vi "initialise.vi"(8 "error in (no error)":errorcluster, 10 "main_app_instance":bool, 11 "Pixelfly in":refnum<class "PixelflySA.lvclass">) -> (0 "error out":errorcluster, 3 "Pixelfly out":refnum<class "PixelflySA.lvclass">)   [LabVIEW 2011, in "PixelflySA.lvclass"]
uses:
  PixelflySA.lvclass
  PixelflySA.lvclass/PixelflySA.ctl
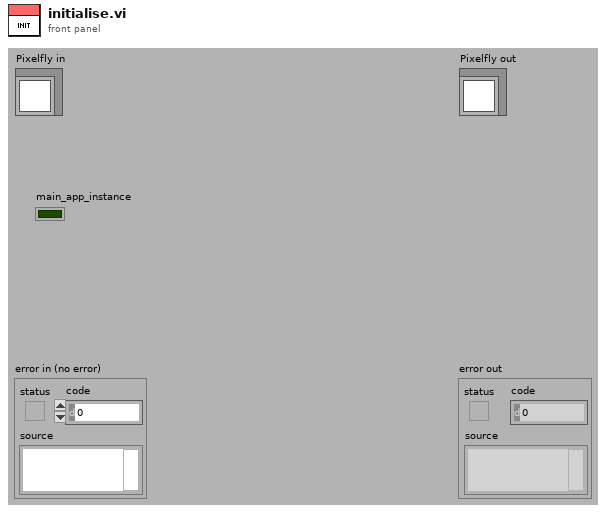
[diagram p1: front panel]
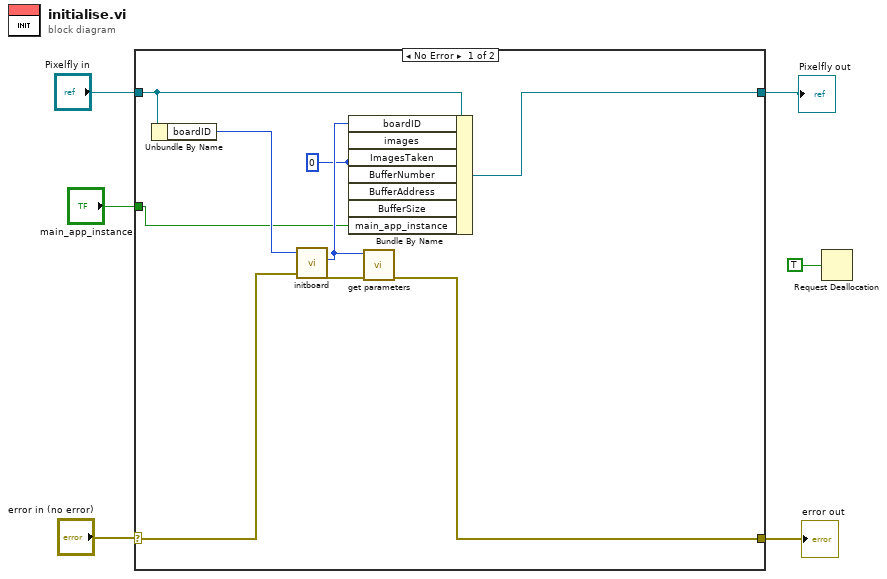
[diagram p0: block diagram]
diagram:
  n1 = case shown="No Error" "error in (no error)" {
    selector: "error in (no error)" -> [w12 w16]
    tunnel: "Pixelfly in" -> [w11 w17]
    tunnel: [w9 w17] -> w4
    tunnel: [w8 w16] -> w3
    tunnel: "main_app_instance" -> [w7 _]
    frame No Error {
      w10 = 0
      n2 = Unbundle By Name(w11) -> ("boardID"=w14:i32)
      n3 = call <instrlib>:"initboard.vi"("boardid in"=w14, "error in (no error)"=w12) -> ("boardid"=w13:i32, "error out"=w15:errorcluster)  [unwired: 2 in, 1 out]
      n4 = Bundle By Name(cluster=w11, "boardID"=w13, "images"=w10, "ImagesTaken"=w10, "BufferNumber"=w10, "BufferAddress"=w10, "BufferSize"=w10, "main_app_instance"=w7) -> (w9:refnum<class "PixelflySA.lvclass">)
      n5 = call <instrlib>:"get parameters.vi"("error in (no error)"=w15, "Handle in"=w13) -> ("error out"=w8:errorcluster)  [unwired: 2 in, 3 out]
    }
    frame Error {
    }
  }
  "error out" <- w3
  "Pixelfly out" <- w4
  n6 = Request Deallocation(TRUE ("flag")) -> ()
